vi "Initialization VI.vi"(8 "error in (no error)":errorcluster, 10 "Custom XML":string, 11 "Device Item Ref in":T1 format="%.0x") -> (0 "error out":errorcluster, 3 "Device Item Ref out":T1 format="%.0x")   [LabVIEW 2017, in "NI-XNET Monitor System Explorer.lvlib"]
uses:
  NI-XNET Monitor System Explorer.lvlib
  <vilib>/NI Veristand/Custom Device API/Custom Device Item Ref.ctl
  Shared/Constants.vi
  Shared/NI-XNET Monitor Shared.lvlib
  <vilib>/NI Veristand/Custom Device API/Custom Device API.lvlib
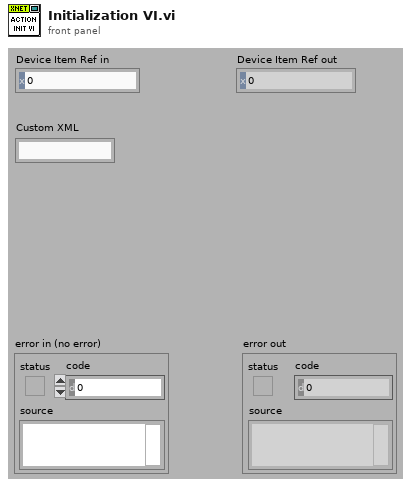
[diagram p1: front panel]
types:
  T1 = typedef "Custom Device API.lvlib/Custom Device Item Ref.ctl" = u64
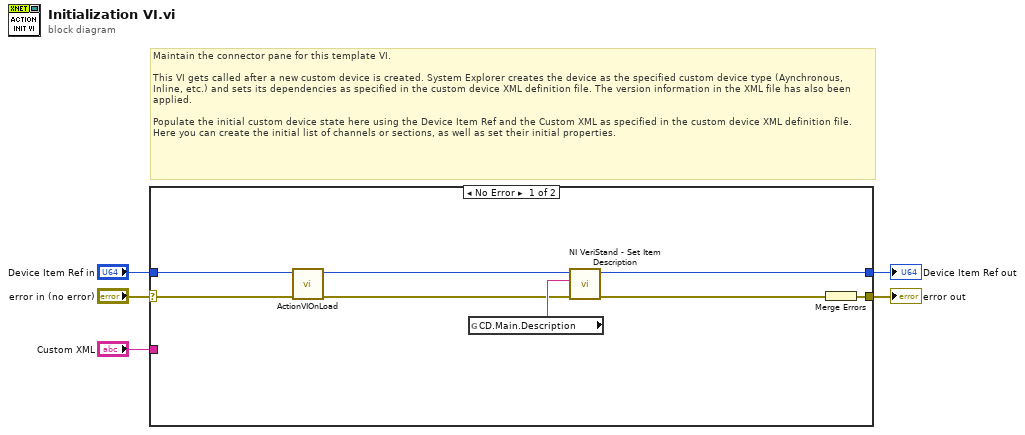
[diagram p0: block diagram]
diagram:
  # "Maintain the connector pane for this template VI.\n\nThis VI gets called after a new custom device is created. System Explorer creates the device as the specified custom device type (Aynchronous, Inline, etc.) and sets its dependencies as specified in the custom device XML definition file. The version information in the XML file has also been applied.\n\nPopulate the initial custom device state here using the Device Item Ref and the Custom XML as specified in the custom device XML definition file. Here you can create the initial list of channels or sections, as well as set their initial properties."
  n1 = case shown="No Error" "error in (no error)" {
    selector: "error in (no error)" -> [w7 w15]
    tunnel: [w10 w15] -> w1
    tunnel: [w13 w14] -> w2
    tunnel: "Device Item Ref in" -> [w9 w14]
    tunnel: "Custom XML" -> [_ _]
    frame No Error {
      n2 = call "ActionVIOnLoad.vi"("Error In"=w7, "Device Item Ref In"=w9) -> ("Error Out"=w6:errorcluster, "Device Item Ref out"=w8:T1)  [unwired: 8 in]
      n3 = global read "Constants.vi" "CD.Main.Description"() -> (w11:string)
      n4 = call <vilib>:"NI VeriStand - Set Item Description.vi"("error in (no error)"=w6, "Description"=w11, "Item Ref in"=w8) -> ("error out"=w12:errorcluster, "Item Ref out"=w13:T1)  [unwired: 6 in, 1 out]
      n5 = Merge Errors(w12) -> (w10:errorcluster)
    }
    frame Error {
    }
  }
  "error out" <- w1
  "Device Item Ref out" <- w2
